vi "AskQuestionToDevice .vi"(11 "ClusterNameDevices":cluster{"Commutator34980A":string}={"Commutator34980A"="34980"}) -> (0 "error out":errorcluster, 3 "ClusterAdresDevices":T1)   [LabVIEW 2017]
uses:
  <vilib>/Instr/_visa.llb/VISA Find Search Mode.ctl
panel:
  out "return count":u32
  out "find list":string[](array[string])
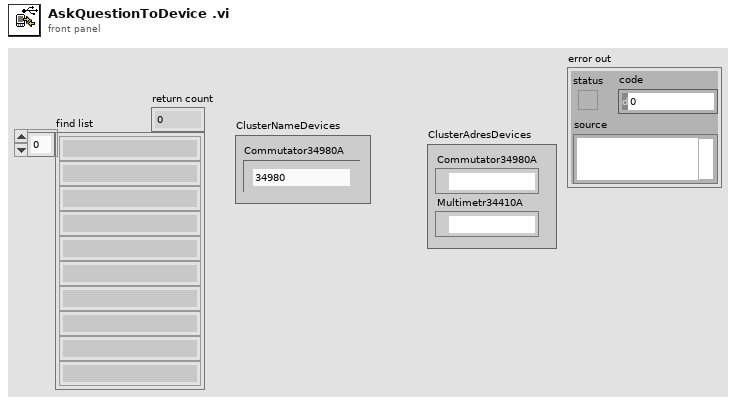
[diagram p1: front panel]
types:
  T1 = cluster{"Commutator34980A":refnum<visa-resource-name>, "Multimetr34410A":refnum<visa-resource-name>}
  T2 = typedef "VISA Find Search Mode.ctl" = u32
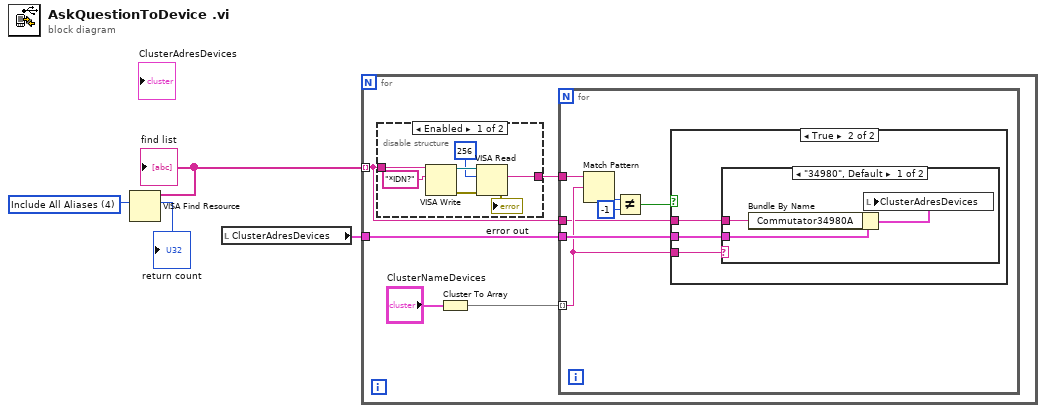
[diagram p0: block diagram]
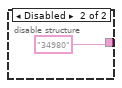
[diagram p2: hidden frame]
diagram:
  w4 = T2 4 items=["Canonical Names Only"=0, "Aliases Only"=2, "Include Matching Aliases"=3, "Include All Aliases"=4] ("Search Mode")
  n1 = VISA Find Resource(10:w4) -> (2:→"return count":u32, 3:w2:string[])  [unwired: 2 in, 1 out]
  "find list" <- w2
  n2 = local read "ClusterAdresDevices"() -> (w1:T1)
  n3 = for {
    tunnel: w2 -> [w5] mode=indexing
    tunnel: w1 -> [w6]
    n4 = disable-structure shown="Enabled" {
      disable-tunnel: w5 -> [w16 _]
      disable-tunnel: [w11 "34980"] -> w7
      frame Enabled {
        n5 = VISA Write(VISA resource name=w16, write buffer="*IDN?" ("ID Query")) -> (VISA resource name out=w13:refnum<visa-resource-name>, error out=w14:errorcluster)  [unwired: 1 in, 1 out]
        n6 = VISA Read(VISA resource name=w13, byte count=u32 256, error in (no error)=w14) -> (read buffer=w11:string, error out=→"error out":errorcluster)  [unwired: 2 out]
      }
      frame Disabled {
      }
    }
    n7 = Cluster To Array(cluster="ClusterNameDevices") -> (array=w8:string[])
    n8 = for {
      tunnel: w7 -> [w24]
      tunnel: w8 -> [w19] mode=indexing
      tunnel: w6 -> [w20]
      tunnel: w5 -> [w18]
      n9 = Match Pattern(string=w24, regular expression=w19) -> (offset past match=w23:i32)  [unwired: 1 in, 3 out]
      n10 = Not Equal?(x=w23, y=-1) -> (x != y?=w21:bool)
      n11 = case shown="True" w21 {
        tunnel: w20 -> [_ w26]
        tunnel: w19 -> [_ w27]
        tunnel: w18 -> [_ w25]
        frame False {
        }
        frame True {
          n12 = case shown="\"34980\", Default" w27 {
            tunnel: w26 -> [w30 _]
            tunnel: w25 -> [w28 _]
            frame "34980", Default {
              n13 = Bundle By Name(cluster=w30, "Commutator34980A"=w28) -> (w29:T1)
              n14 = local write "ClusterAdresDevices"(w29) -> ()
            }
            frame "True" {
            }
          }
        }
      }
    }
  }
